vi "JSONRPC-ArrayToString_Cluster.vi"(11 "List":T1(array[cluster])) -> (3 "Output":string)   [LabVIEW 2020]
panel:
  # "ArrayToString_Cluster"
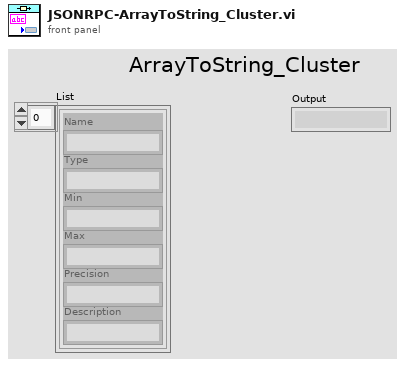
[diagram p1: front panel]
types:
  T1 = cluster{"Name":string, "Type":string, "Min":string, "Max":string, "Precision":string, "Description":string}[]
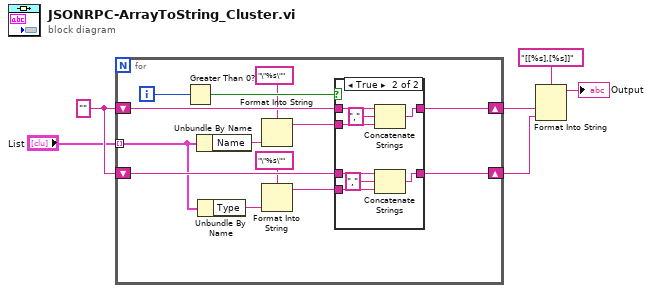
[diagram p0: block diagram]
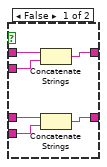
[diagram p2: hidden frame]
diagram:
  w2 = ""
  n1 = for {
    tunnel: "List" -> [w13] mode=indexing
    shift-right: [w19] -> w6
    shift-left: w2 -> [w18]
    shift-right: [w15] -> w5
    shift-left: w2 -> [w14]
    i -> [w17]
    n2 = Greater Than 0?(x=w17) -> (x > 0?=w16:bool)
    n3 = Unbundle By Name(w13) -> ("Name"=w11:string)
    n4 = Unbundle By Name(w13) -> ("Type"=w8:string)
    n5 = Format Into String(format string="\"%s\"", w11) -> (resulting string=w10:string)  [unwired: 2 in, 1 out]
    n6 = Format Into String(format string="\"%s\"", w8) -> (resulting string=w7:string)  [unwired: 2 in, 1 out]
    n7 = case shown="True" w16 {
      tunnel: w10 -> [w25 w32]
      tunnel: [w24 w33] -> w19
      tunnel: w18 -> [w23 w31]
      tunnel: w7 -> [w22 w27]
      tunnel: [w21 w26] -> w15
      tunnel: w14 -> [w20 w28]
      frame False {
        n8 = Concatenate Strings(w23, w25) -> (w24:string)
        n9 = Concatenate Strings(w20, w22) -> (w21:string)
      }
      frame True {
        n10 = Concatenate Strings(w31, ",", w32) -> (w33:string)
        n11 = Concatenate Strings(w28, ",", w27) -> (w26:string)
      }
    }
  }
  n12 = Format Into String(format string="[[%s],[%s]]", w6, w5) -> (resulting string=→"Output":string)  [unwired: 2 in, 1 out]
